vi "plot_usr_seq2.vi"(1 "User-defined sequence":string[][](table)) -> (0 "Waveform Chart":cluster{dbl, dbl, dbl}(graph))   [LabVIEW 2014]
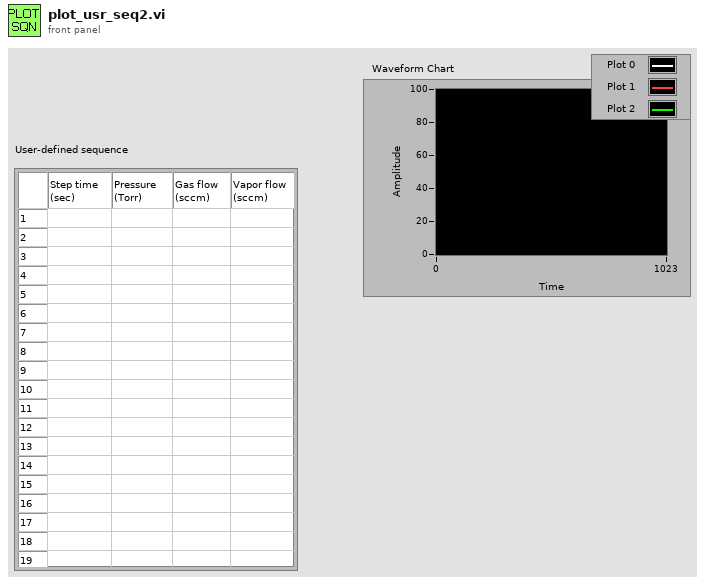
[diagram p1: front panel]
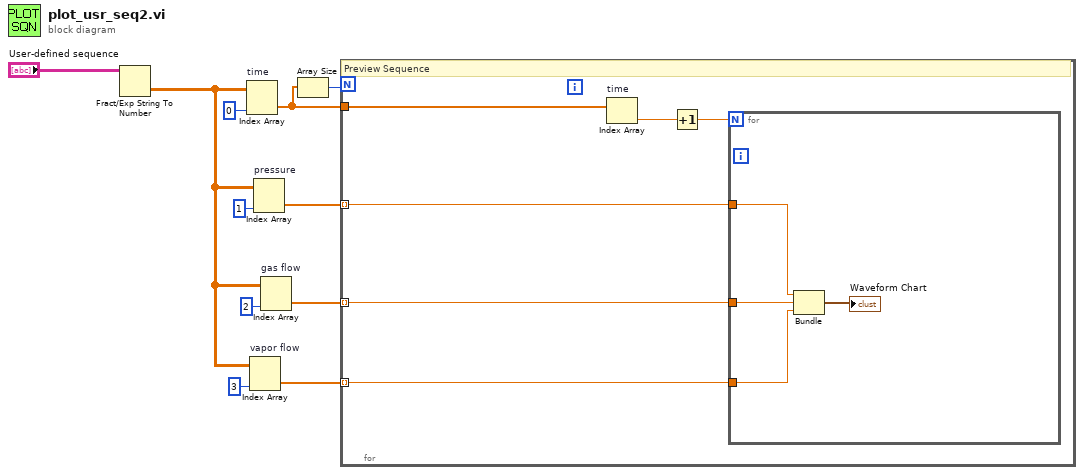
[diagram p0: block diagram]
diagram:
  n1 = Fract/Exp String To Number(string="User-defined sequence") -> (number=w3:dbl[][])  [unwired: 3 in, 1 out]
  n2 = Index Array "time"(array=w3, index (col)=0 ("disabled index (col)")) -> (element=w7:dbl[])  [unwired: 1 in]
  n3 = Index Array "vapor flow"(array=w3, index (col)=3 ("disabled index (col)")) -> (element=w1:dbl[])  [unwired: 1 in]
  n4 = Index Array "pressure"(array=w3, index (col)=1 ("disabled index (col)")) -> (element=w8:dbl[])  [unwired: 1 in]
  n5 = Index Array "gas flow"(array=w3, index (col)=2 ("disabled index (col)")) -> (element=w2:dbl[])  [unwired: 1 in]
  n6 = Array Size(array=w7) -> (size(s)=w6:i32)
  n7 = for {
    N: w6 -> [_]
    tunnel: w7 -> [w17]
    tunnel: w8 -> [w13] mode=indexing
    tunnel: w2 -> [w12] mode=indexing
    tunnel: w1 -> [w14] mode=indexing
    # "Preview Sequence"
    n8 = Index Array "time"(array=w17) -> (element=w16:dbl)  [unwired: 1 in]
    n9 = Increment(x=w16) -> (x+1=w15:dbl)
    n10 = for {
      N: w15 -> [_]
      tunnel: w13 -> [w20]
      tunnel: w12 -> [w19]
      tunnel: w14 -> [w18]
      n11 = Bundle(w20, w19, w18) -> (→"Waveform Chart":cluster{dbl, dbl, dbl})  [unwired: 1 in]
    }
  }
